vi "pEnable to U32.vi"(2 "pEnable":T1) -> (16 "pEnable out":u32)   [LabVIEW 2013, in "VRI.lvlib"]
uses:
  VRI.lvlib
  _Type Defs/pEnable.ctl
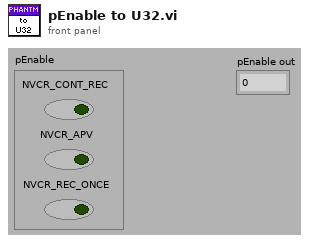
[diagram p1: front panel]
types:
  T1 = typedef "VRI.lvlib/pEnable.ctl" = cluster{"NVCR_CONT_REC":bool, "NVCR_APV":bool, "NVCR_REC_ONCE":bool}
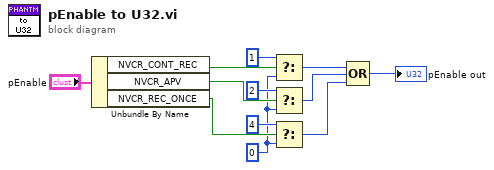
[diagram p0: block diagram]
diagram:
  w5 = u32 0 ("f")
  n1 = Unbundle By Name("pEnable") -> ("NVCR_CONT_REC"=w11:bool, "NVCR_APV"=w10:bool, "NVCR_REC_ONCE"=w9:bool)
  n2 = Select(t=u32 1, s=w11, f=w5) -> (s? t:f=w4:u32)
  n3 = Select(t=u32 2, s=w10, f=w5) -> (s? t:f=w3:u32)
  n4 = Select(t=u32 4, s=w9, f=w5) -> (s? t:f=w2:u32)
  n5 = Compound Arithmetic op=OR(w4, w3, w2) -> (→"pEnable out":u32)
